vi "Locate Subset by Code.vi"(7 "Read channels":string[](array[string]), 8 "error in":errorcluster, 9 "Start":i64, 10 "Start code":i32=6, 11 "File Path":path=path "C:/Data/October_2025/102525/m003_111527_102525.tdms") -> (0 "error out":errorcluster={"status"=TRUE, "code"=-2532, "source"="TDMS Read in loacate subset.vi"}, 1 "Length out":i32, 2 "End Index out":i32=-1, 3 "file path out":path=path "\\\\myhome\\NHMFL/Projects/Pressure/Code/Alex/m006_092123.tdms", 5 "Data out":dbl[][](array[numeric]), 6 "Start Index out":i32=-1)   [LabVIEW 2024]
panel:
  in  "Status  Channel":string="B status"
  in  "End code":i32=5
  out "Waveform Graph 2":dbl[](graph)
  out "Waveform Graph":waveform(dbl)[](graph)
  in  "group name in":string="p"
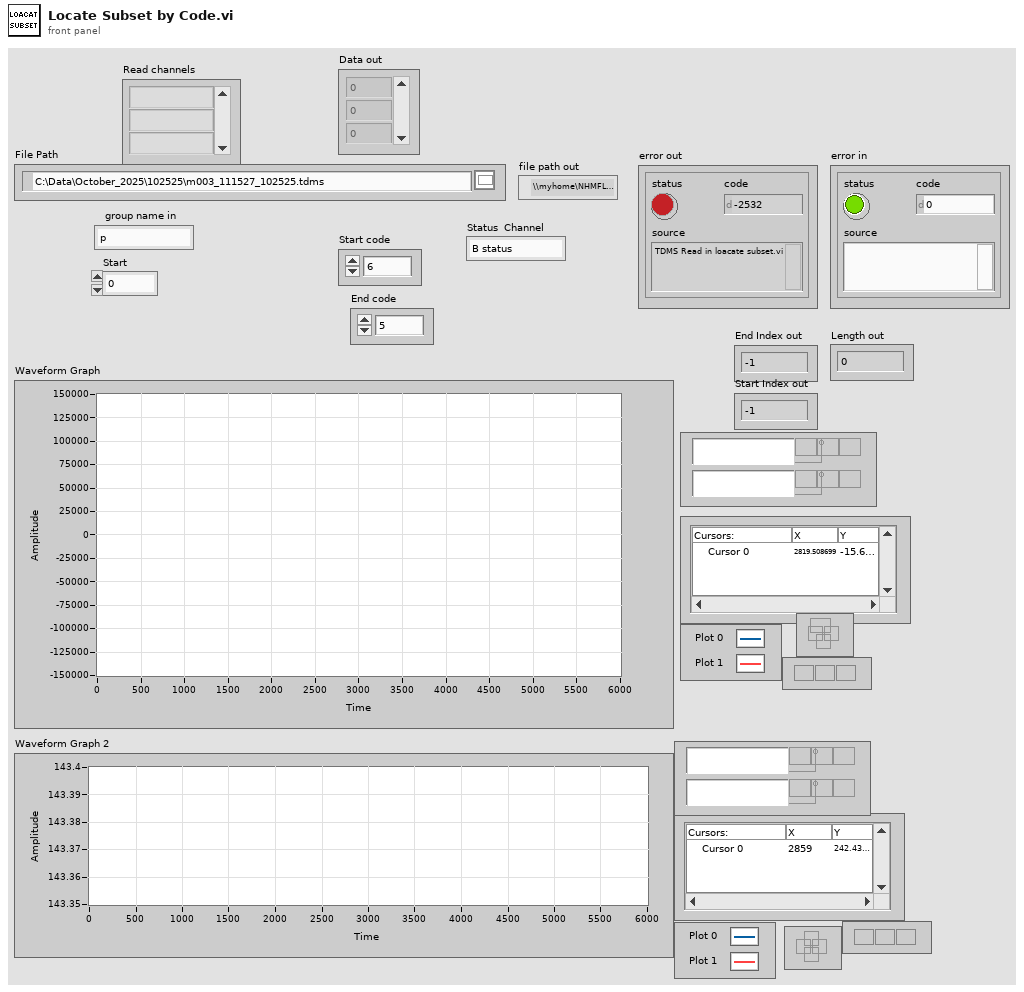
[diagram p1: front panel]
types:
  T1 = enum16{"open", "open or create", "create or replace", "create", "open (read-only)"}
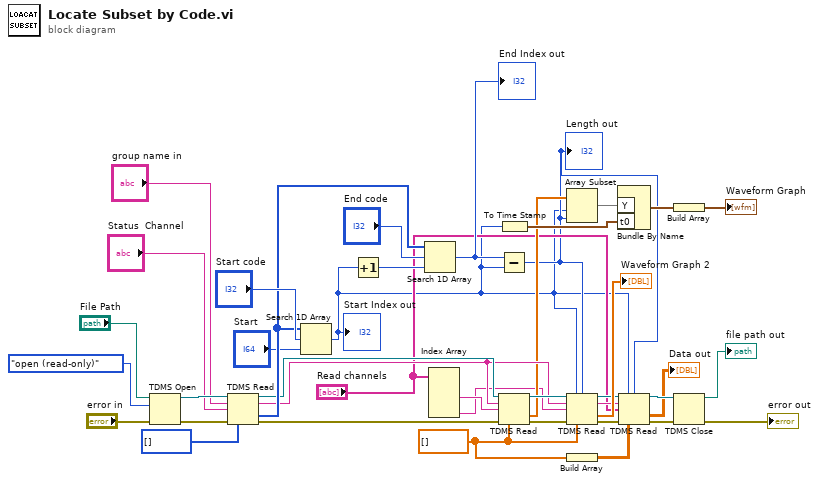
[diagram p0: block diagram]
diagram:
  w8 = dbl[] []
  n1 = TDMS Open(8:"error in", 10:T1."open (read-only)" ("operation (0:open)"), 11:"File Path") -> (0:w38:errorcluster, 3:w39:refnum<k34>)  [unwired: 4 in]
  n2 = TDMS Read(0:w39, 5:"group name in", 7:"Status  Channel", 11:w38, 12:i32[] []) -> (4:w21:refnum<k34>, 6:w18:string, 10:w25:i32[], 15:w22:errorcluster)  [unwired: 3 in, 2 out]
  n3 = Search 1D Array(1D array=w25, element="Start code", start index (0)="Start") -> (index of element=w1:i32)
  "Start Index out" <- w1
  n4 = Increment(x=w1) -> (x+1=w23:i32)
  n5 = Search 1D Array(1D array=w25, element="End code", start index (0)=w23) -> (index of element=w14:i32)
  "End Index out" <- w14
  n6 = Index Array(array="Read channels") -> (element #2=w4:string, element #4=w3:string)  [unwired: 4 in, 2 out]
  n7 = Subtract(x=w14, y=w1) -> (x-y=w2:i32)
  "Length out" <- w2
  n8 = TDMS Read(0:w21, 5:w18, 7:w4, 11:w22, 12:w8) -> (4:w20:refnum<k34>, 10:w17:dbl[], 15:w19:errorcluster)  [unwired: 3 in, 3 out]
  n9 = To Time Stamp(1:w1) -> (0:w27:timestamp)
  n10 = Array Subset(array=w17, index=w1, length=w2) -> (w30:dbl[])
  n11 = TDMS Read(0:w20, 1:w1, 2:w2, 5:w18, 7:w3, 11:w19, 12:w8) -> (4:w10:refnum<k34>, 6:w11:string, 10:→"Waveform Graph 2":dbl[], 15:w13:errorcluster)  [unwired: 1 in, 2 out]
  n12 = Build Array(w8) -> (w7:dbl[][])
  n13 = Bundle By Name("Y"=w30, "t0"=w27) -> (w36:waveform(dbl))  [unwired: 1 in]
  n14 = TDMS Read(0:w10, 1:w1, 2:w2, 5:w11, 7:"Read channels", 11:w13, 12:w7) -> (4:w9:refnum<k34>, 10:→"Data out":dbl[][], 15:w12:errorcluster)  [unwired: 1 in, 3 out]
  n15 = Build Array(w36) -> (→"Waveform Graph":waveform(dbl)[])
  n16 = TDMS Close(8:w12, 11:w9) -> (0:→"error out":errorcluster, 3:→"file path out":path)
